vi "Omni-teste-maze.vi"() -> ()   [LabVIEW 2012]
panel:
  in  "stop":bool
  in  "Spectrometer number":i32
  out "Length":i32
  in  "Integration Time (ms)":i32=100
  out "Number of Spectrometers":i32
  out "XY Graph":T1(graph)
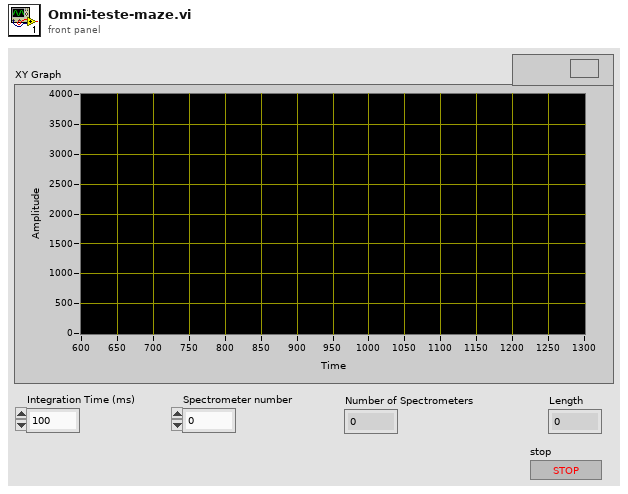
[diagram p1: front panel]
types:
  T1 = cluster{"WL Values":dbl[], "Spectrum Values":dbl[]}
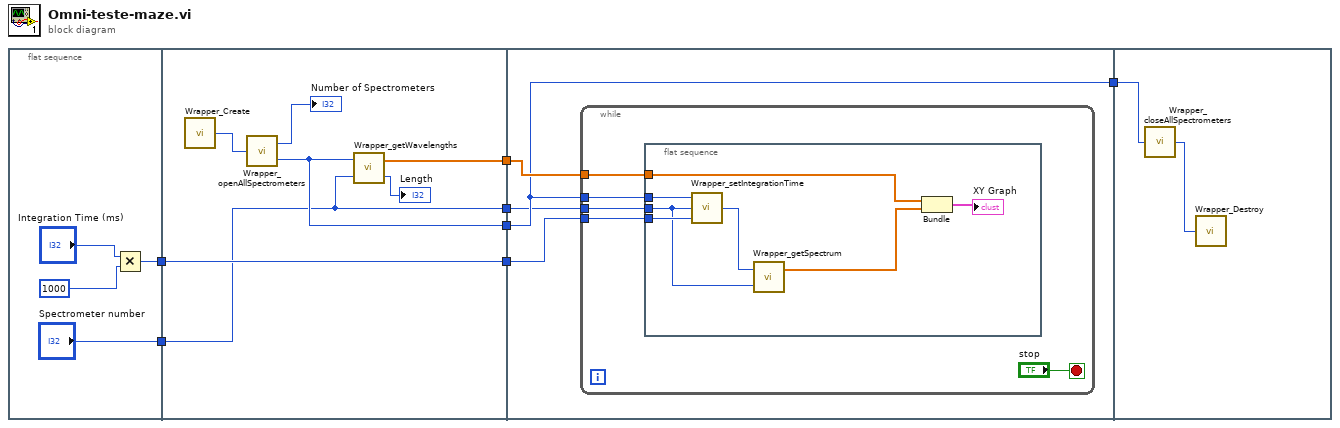
[diagram p0: block diagram]
diagram:
  n1 = flat-sequence {
    tunnel: [w9] -> w5
    tunnel: ["Spectrometer number"] -> w2
    tunnel: [w17] -> w7
    tunnel: [w16] -> w6
    tunnel: w5 -> [w16]
    tunnel: [w14] -> w4
    tunnel: w2 -> [w12]
    tunnel: [w12] -> w1
    tunnel: w7 -> [w22]
    tunnel: w6 -> [w21]
    tunnel: w4 -> [w20]
    tunnel: [w20] -> w3
    tunnel: w1 -> [w19]
    tunnel: w3 -> [w35]
    frame #0 {
      n2 = Multiply(x="Integration Time (ms)", y=1000) -> (x*y=w9:i32)
    }
    frame #1 {
      n3 = call "Wrapper_Create.vi"() -> ("Wrapper"=w13:u32)
      n4 = call "Wrapper_openAllSpectrometers.vi"("Wrapper In"=w13) -> ("Number of Spectrometers"=→"Number of Spectrometers":i32, "Wrapper Out"=w14:u32)
      n5 = call "Wrapper_getWavelengths.vi"("Index"=w12, "Wrapper"=w14) -> ("Length"=→"Length":i32, "WL Values"=w17:dbl[])
    }
    frame #2 {
      n6 = while {
        tunnel: w22 -> [w27]
        tunnel: w21 -> [w26]
        tunnel: w20 -> [w25]
        tunnel: w19 -> [w24]
        stop <- "stop" stop-if-true
        n7 = flat-sequence {
          tunnel: w27 -> [w34]
          tunnel: w26 -> [w30]
          tunnel: w25 -> [w29]
          tunnel: w24 -> [w28]
          frame #0 {
            n8 = call "Wrapper_setIntegrationTime.vi"("Integration Time"=w30, "Index"=w28, "Wrapper In"=w29) -> ("Wrapper Out"=w31:u32)
            n9 = call "Wrapper_getSpectrum.vi"("Index"=w28, "Wrapper"=w31) -> ("Spectrum Values"=w33:dbl[])  [unwired: 1 out]
            n10 = Bundle("WL Values"=w34, "Spectrum Values"=w33) -> (→"XY Graph":T1)  [unwired: 1 in]
          }
        }
      }
    }
    frame #3 {
      n11 = call "Wrapper_closeAllSpectrometers.vi"("Wrapper In"=w35) -> ("Wrapper Out"=w36:u32)
      n12 = call "Wrapper_Destroy.vi"("Wrapper"=w36) -> ()
    }
  }
